vi "HTTP Status Check.vi"(7 "error in (no error)":errorcluster, 10 "String":string) -> (0 "error out":errorcluster, 3 "HTTP Status Code":string)   [LabVIEW 2019, in "DataLogger.lvclass"]
doc: "HTTP Status Check"
uses:
  DataLogger.lvclass
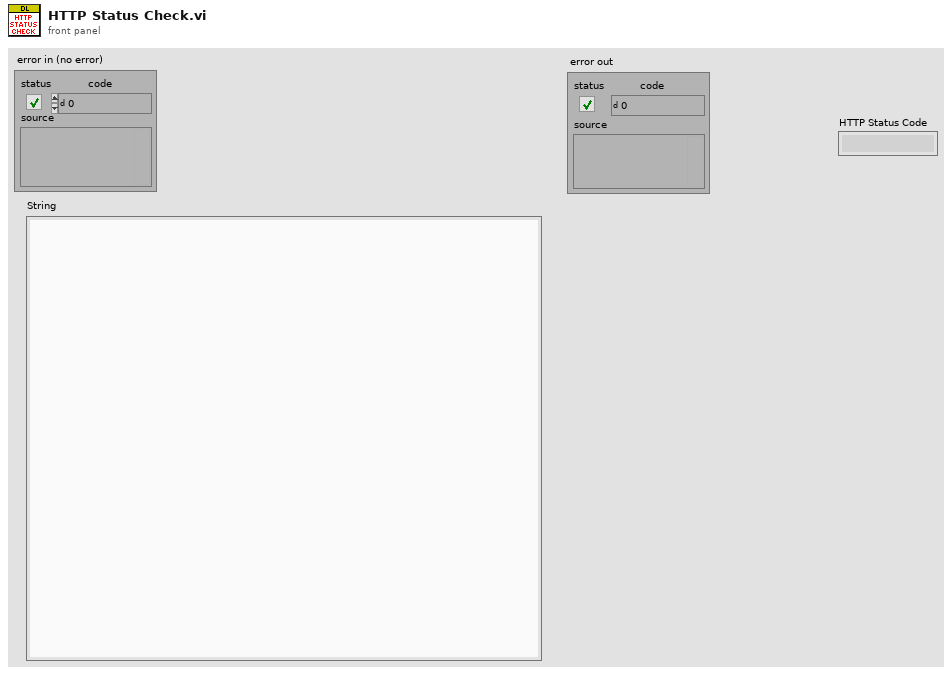
[diagram p1: front panel]
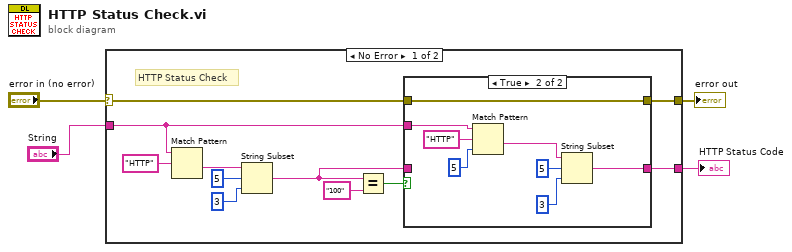
[diagram p0: block diagram]
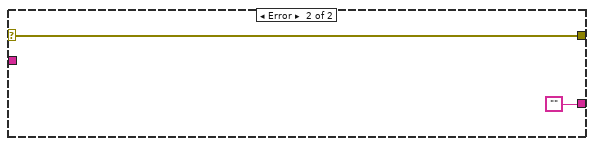
[diagram p3: hidden frame]
diagram:
  n1 = case shown="No Error" "error in (no error)" {
    selector: "error in (no error)" -> [w5 w27]
    tunnel: "String" -> [w11 _]
    tunnel: [w9 w27] -> w3
    tunnel: [w6 ""] -> w2
    frame No Error {
      # "HTTP Status Check"
      n2 = Match Pattern(string=w11, regular expression="HTTP") -> (after substring=w13:string)  [unwired: 1 in, 3 out]
      n3 = String Subset(string=w13, offset (0)=5, length (rest)=3 ("length (rest)")) -> (substring=w8:string)
      n4 = Equal?(x=w8, y="100") -> (x = y?=w10:bool)
      n5 = case shown="True" w10 {
        tunnel: w11 -> [_ w20]
        tunnel: [w17 w18] -> w6
        tunnel: w8 -> [w17 _]
        tunnel: [w16 w19] -> w9
        tunnel: w5 -> [w16 w19]
        frame False {
        }
        frame True {
          n6 = Match Pattern(string=w20, regular expression="HTTP", offset (0)=5) -> (after substring=w23:string)  [unwired: 3 out]
          n7 = String Subset(string=w23, offset (0)=5, length (rest)=3 ("length (rest)")) -> (substring=w18:string)
        }
      }
    }
    frame Error {
    }
  }
  "error out" <- w3
  "HTTP Status Code" <- w2
